vi "Destroy Notifiers.vi"(8 "error in (no error)":errorcluster, 11 "Transport in":refnum<class "Transport.lvclass">) -> (0 "error out":errorcluster)   [LabVIEW 2019, in "Transport.lvclass"]
uses:
  Transport.lvclass
  Transport.lvclass/Transport.ctl
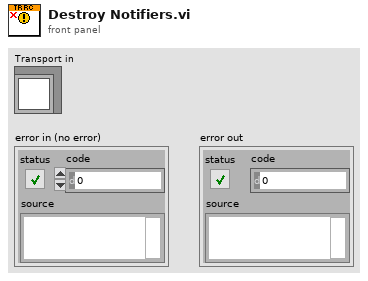
[diagram p1: front panel]
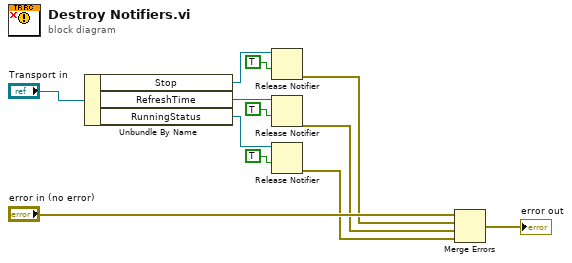
[diagram p0: block diagram]
diagram:
  n1 = Unbundle By Name("Transport in") -> ("Stop"=w11:refnum<notifier>, "RefreshTime"=w8:refnum<notifier>, "RunningStatus"=w6:refnum<notifier>)
  n2 = Release Notifier(notifier=w11, force destroy? (F)=TRUE) -> (error out=w4:errorcluster)  [unwired: 1 in, 2 out]
  n3 = Release Notifier(notifier=w8, force destroy? (F)=TRUE) -> (error out=w3:errorcluster)  [unwired: 1 in, 2 out]
  n4 = Release Notifier(notifier=w6, force destroy? (F)=TRUE) -> (error out=w2:errorcluster)  [unwired: 1 in, 2 out]
  n5 = Merge Errors("error in (no error)", w4, w3, w2) -> (→"error out":errorcluster)
